vi "Strings1.vi"() -> ()   [LabVIEW 2020]
panel:
  out "result string":string
  in  "length (len. of substring)":i32
  in  "offset (0)":i32
  in  "substring (\"\")":string
  in  "string 2":string
  out "concatenated string":string
  out "length":i32
  in  "string":string
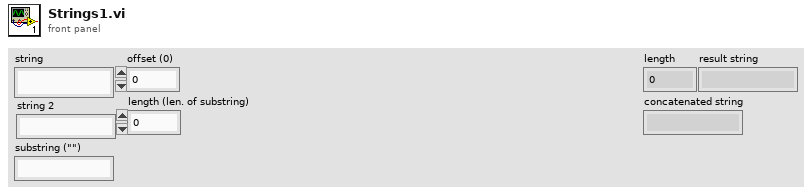
[diagram p1: front panel]
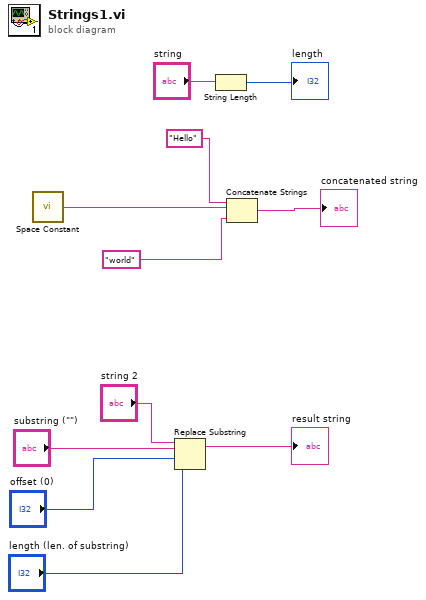
[diagram p0: block diagram]
diagram:
  n1 = call <vilib>:"Space Constant.vi"() -> ("String"=w6:string)
  n2 = Replace Substring(2:"length (len. of substring)", 3:"offset (0)", 4:"substring (\"\")", 5:"string 2") -> (1:→"result string":string)  [unwired: 1 out]
  n3 = String Length(string="string") -> (length=→"length":i32)
  n4 = Concatenate Strings("Hello" ("string"), w6, "world" ("string")) -> (→"concatenated string":string)
